vi "KeepGoingUntilPosReached.vi"(7 "Variables d'Axes":T1={"OrdreBloc"="ni.var.psp://localhost/OPC/OPC1/esbimETH_1/module1/2AXBOC/E0_Ordre/Axe2_OrdreBloc", "Ordre UC"="ni.var.psp://localhost/OPC/OPC1/esbimETH_1/module1/2AXBOC/E0_Ordre/Axe2_OrdreUC", "CoteAAtteindre"="ni.var.psp://localhost/OPC/OPC1/esbimETH_1/module1/2AXBOC/E2_Position2/CoteAAtteindre", "Vitesse"="ni.var.psp://localhost/OPC/OPC1/esbimETH_1/module1/2AXBOC/E2_Position2/Vitesse", "Position codeur en pas"="ni.var.psp://localhost/OPC/OPC1/esbimETH_1/module1/2AXBOC/L4_PositionPas/Axe2_PositionCodeurEnPas", "Position Théorique"="ni.var.psp://localhost/OPC/OPC1/esbimETH_1/module1/2AXBOC/L0_Position/Axe2_PositionTheorique", "Message"="ni.var.psp://localhost/OPC/OPC1/esbimETH_1/module1/2AXBOC/L0_Position/Axe2_Messages", "Ecrire"="ni.var.psp://localhost/OPC/OPC1/esbimETH_1/module1/2AXBOC/ecrire", "Zone à écrire"="ni.var.psp://localhost/OPC/OPC1/esbimETH_1/module1/2AXBOC/zones_a_ecrire", "Numéro paramètre"="ni.var.psp://localhost/OPC/OPC1/esbimETH_1/module1/2AXBOC/E3_Parametres/NumeroParametre", "Ordre"="ni.var.psp://localhost/OPC/OPC1/esbimETH_1/module1/2AXBOC/E3_Parametres/Ordre", "Valeur"="ni.var.psp://localhost/OPC/OPC1/esbimETH_1/module1/2AXBOC/E3_Parametres/Valeur", "Valeur Lecture"="ni.var.psp://localhost/OPC/OPC1/esbimETH_1/module1/2AXBOC/L2_Parametres/Valeur", "Numéro paramètre Lecture"="ni.var.psp://localhost/OPC/OPC1/esbimETH_1/module1/2AXBOC/L2_Parametres/Numero", "Acquittement Lecture Ecriture"="ni.var.psp://localhost/OPC/OPC1/esbimETH_1/module1/2AXBOC/L2_Parametres/AcquitementLectureEcriture", "Zone à Ecrire Pour Axe "=0, "Acquittement Ordre UC"=""}, 8 "error in (no error)":errorcluster caption="entrée d'erreur (pas d'erreur)", 9 "Cote à atteindre":i32, 10 "Axe?":enum16{"Axe1", "Axe2", "Axe3"}(ring)) -> (0 "error out":errorcluster caption="sortie d'erreur", 1 "Nombre d'essais":i32)   [LabVIEW 2013]
uses:
  Commandes/Type de Mouvement PilMOT.ctl
  Controls/AdressesVariablesPartagees.ctl
panel:
  in  "Axe3_PositionTheorique":i32
  in  "Axe2_PositionCodeurEnPas 2":i32
  in  "Axe1_PositionTheorique":i32
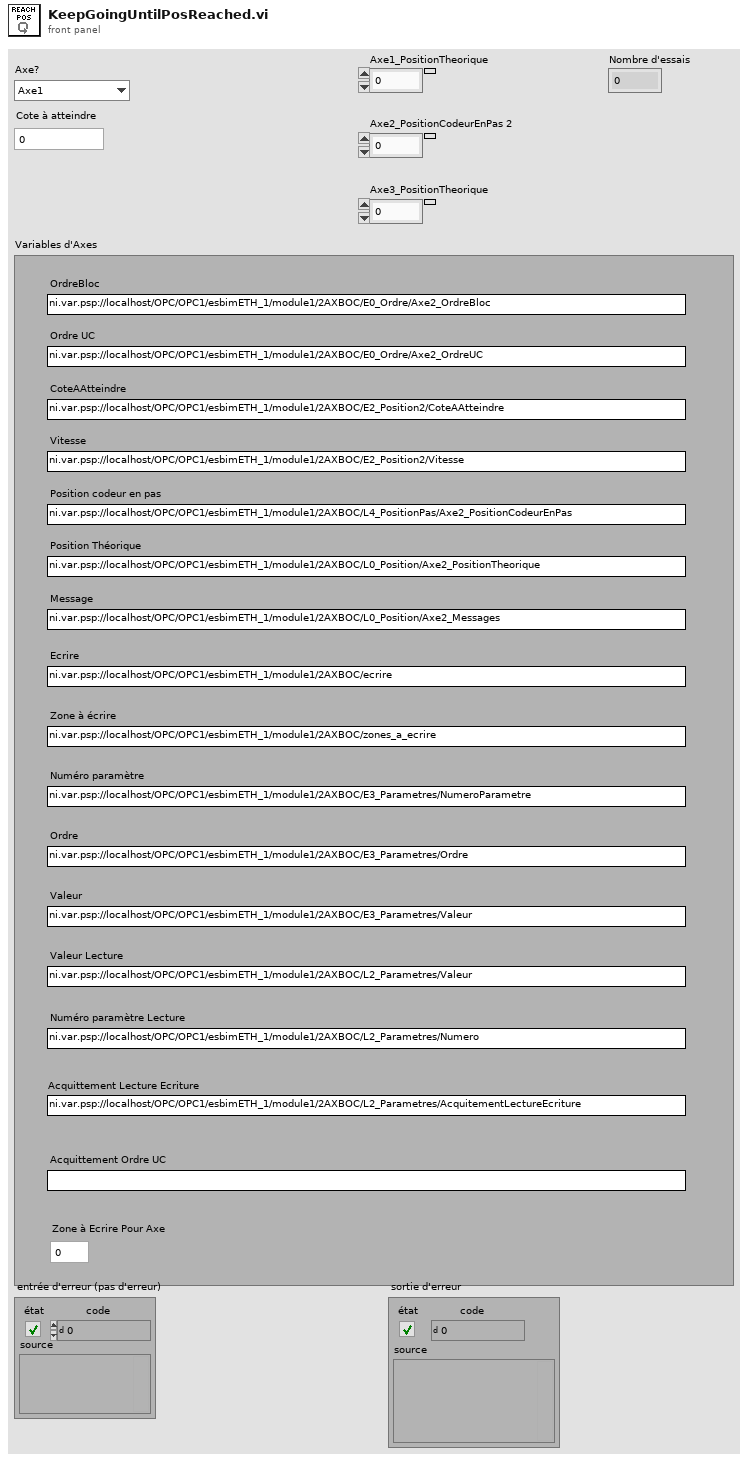
[diagram p1: front panel]
types:
  T1 = typedef "AdressesVariablesPartagees.ctl" = cluster{"OrdreBloc":string, "Ordre UC":string, "CoteAAtteindre":string, "Vitesse":string, "Position codeur en pas":string, "Position Théorique":string, "Message":string, "Ecrire":string, "Zone à écrire":string, "Numéro paramètre":string, "Ordre":string, "Valeur":string, "Valeur Lecture":string, "Numéro paramètre Lecture":string, "Acquittement Lecture Ecriture":string, "Zone à Ecrire Pour Axe ":u16, "Acquittement Ordre UC":string}
  T2 = typedef "Type de Mouvement PilMOT.ctl" = u16
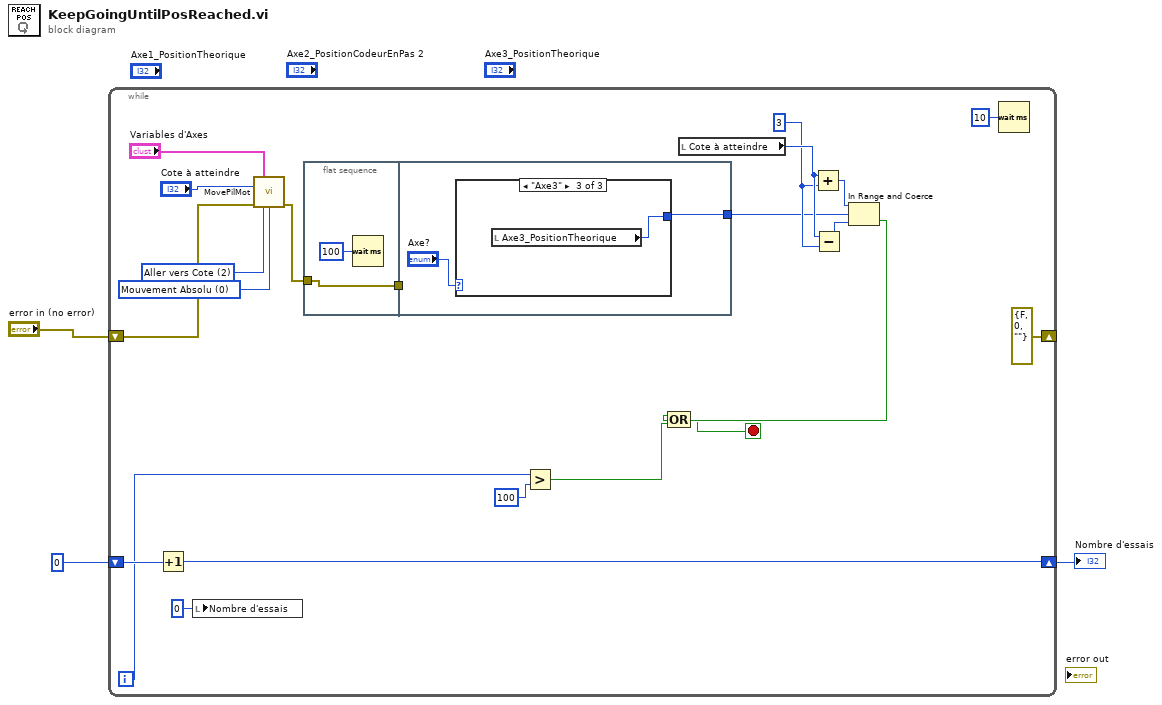
[diagram p0: block diagram]
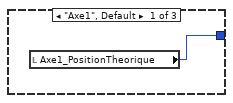
[diagram p2: hidden frame]
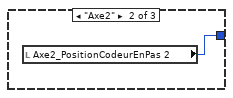
[diagram p3: hidden frame]
diagram:
  n1 = while {
    shift-right: [errorcluster {"status"=FALSE, "code"=0, "source"=""} ("error in (no error)")] -> _
    shift-left: "error in (no error)" -> [w24]
    shift-right: [w16] -> w1
    shift-left: 0 -> [w17]
    i -> [w7]
    stop <- w8 stop-if-true
    w11 = 3 ("Cote à atteindre")
    w22 = u16 0 items=["Mouvement Relatif"=1, "Mouvement Absolu"=0] ("Mouvement Absolu/Relatif")
    w23 = T2 2 items=["Mouvement Simple"=1, "Aller vers Cote"=2, "Va vers position de référence"=3] ("Type de mouvement")
    n2 = Increment(x=w17) -> (x+1=w16:i32)
    n3 = local write "Nombre d'essais"(0 ("Nombre d'essais")) -> ()
    n4 = call "MovePilMot.vi"("Variables d'Axes"="Variables d'Axes", "Cote à atteindre"="Cote à atteindre", "error in (no error)"=w24, "Type de mouvement"=w23, "Mouvement Absolu/Relatif"=w22) -> ("error out"=w20:errorcluster)  [unwired: 10 in]
    n5 = flat-sequence {
      tunnel: w20 -> [w26]
      tunnel: [w26] -> w5
      tunnel: w5 -> [_]
      tunnel: [w28] -> w4
      frame #0 {
        n6 = Wait (ms)(milliseconds to wait=u32 100 ("attente (ms)")) -> ()  [unwired: 1 out]
      }
      frame #1 {
        n7 = case shown="\"Axe3\"" "Axe?" {
          tunnel: [w30 w31 w32] -> w28
          frame "Axe1", Default {
            n8 = local read "Axe1_PositionTheorique"() -> (w30:i32)
          }
          frame "Axe2" {
            n9 = local read "Axe2_PositionCodeurEnPas 2"() -> (w31:i32)
          }
          frame "Axe3" {
            n10 = local read "Axe3_PositionTheorique"() -> (w32:i32)
          }
        }
      }
    }
    n11 = Greater?(x=w7, y=100 ("x")) -> (0:w19:bool)
    n12 = local read "Cote à atteindre"() -> (w12:i32)
    n13 = Add(x=w12, y=w11) -> (x+y=w14:i32)
    n14 = Subtract(x=w12, y=w11) -> (x-y=w13:i32)
    n15 = In Range and Coerce(upper limit=w14, x=w4, lower limit=w13) -> (In Range?=w10:bool)  [unwired: 1 out]
    n16 = Compound Arithmetic op=OR(w10, w19) -> (w8:bool)
    n17 = Wait (ms)(milliseconds to wait=u32 10) -> ()  [unwired: 1 out]
  }
  "Nombre d'essais" <- w1
